vi "Get Sparse Marker Indexes [SM].vi"(8 "error in (no error)":errorcluster, 9 "Marker Name (\"\")":string caption="marker name (\"\")", 10 "Indexes Array Size":i64 caption="indexes array size" format="%.0g", 11 "CS++Fgen in":refnum<class "CS++Fgen.lvclass">) -> (0 "error out":errorcluster, 1 "Indexes Array":i64[](array[numeric]) caption="indexes array", 2 "Indexes Actual Size":i64 caption="indexes actual size", 3 "CS++Fgen out":refnum<class "CS++Fgen.lvclass">)   [LabVIEW 2013, in "CS++Fgen.lvlib" / "CS++Fgen.lvclass"]
doc: "The VI returns the coerced indexes associated with the sparse marker. You can use the following VIs to specify indexes:\n\n- IviFgen Configure Sparse Marker [SM] VI\n- IviFgen Set Sparse Marker Indexes [SM] VI\n\nNote:\n\n(1) This VI is part of the IviFgenSparseMarker [SM] extension group."
uses:
  CS++Fgen.lvclass
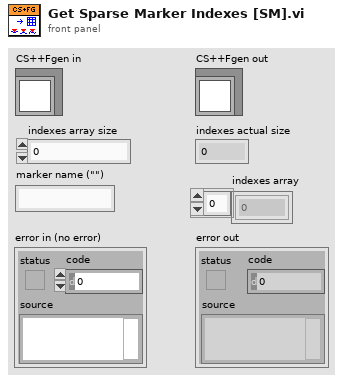
[diagram p1: front panel]
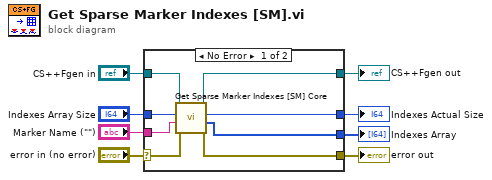
[diagram p0: block diagram]
diagram:
  n1 = case shown="No Error" "error in (no error)" {
    selector: "error in (no error)" -> [w13 w18]
    tunnel: [w12 w18] -> w7
    tunnel: [w15 w17] -> w5
    tunnel: "CS++Fgen in" -> [w16 w17]
    tunnel: "Marker Name (\"\")" -> [w11 _]
    tunnel: "Indexes Array Size" -> [w14 _]
    tunnel: [w10 _] -> w2
    tunnel: [w9 _] -> w1
    frame No Error {
      n2 = call-dynamic "Get Sparse Marker Indexes [SM] Core.vi"("error in (no error)"=w13, "Marker Name (\"\")"=w11, "Indexes Array Size"=w14, "CS++Fgen in"=w16) -> ("error out"=w12:errorcluster, "Indexes Array"=w9:i64[], "Indexes Actual Size"=w10:i64, "CS++Fgen out"=w15:refnum<class "CS++Fgen.lvclass">)  [unwired: 4 in]
    }
    frame Error {
    }
  }
  "error out" <- w7
  "CS++Fgen out" <- w5
  "Indexes Actual Size" <- w2
  "Indexes Array" <- w1
